vi "array - smart min max.vi"(6 "median range":dbl=0.05, 11 "x":dbl[](array[numeric])=[1.0, 5.0, 3.0, 7.0, 0.0]) -> (2 "min":dbl, 3 "max":dbl)   [LabVIEW 2021]
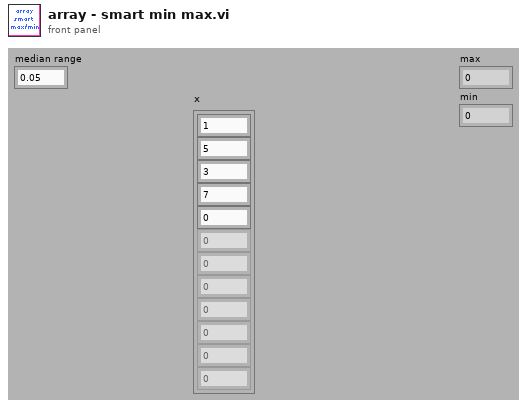
[diagram p1: front panel]
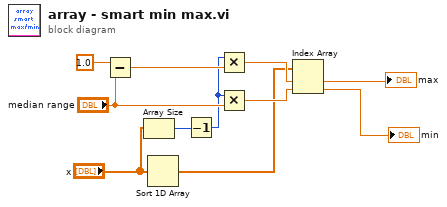
[diagram p0: block diagram]
diagram:
  n1 = Subtract(x=1.0, y="median range") -> (x-y=w8:dbl)
  n2 = Array Size(array="x") -> (size(s)=w2:i32)
  n3 = Sort 1D Array(array="x") -> (sorted array=w5:dbl[])
  n4 = Decrement(x=w2) -> (x-1=w1:i32)
  n5 = Multiply(x=w1, y=w8) -> (x*y=w7:dbl)
  n6 = Multiply(x=w1, y="median range") -> (x*y=w6:dbl)
  n7 = Index Array(array=w5, index #1=w7, index #2=w6) -> (element #1=→"max":dbl, element #2=→"min":dbl)
